vi "GetNumpyExampleModulePath.vi"() -> (3 "module path":path)   [LabVIEW 2023]
doc: "Helper VI to compute the path of the module used by the Python examples."
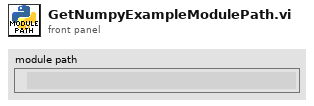
[diagram p1: front panel]
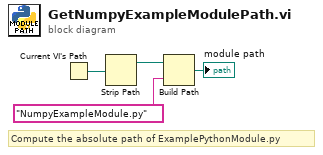
[diagram p0: block diagram]
diagram:
  # "Compute the absolute path of ExamplePythonModule.py"
  n1 = Current VI's Path() -> (path=w4:path)
  n2 = Strip Path(path=w4) -> (stripped path=w3:path)  [unwired: 1 out]
  n3 = Build Path(base path=w3, name or relative path="NumpyExampleModule.py") -> (appended path=→"module path":path)
